vi "Cal.vi"() -> ()   [LabVIEW 2012]
panel:
  in  "3. Next":bool
  out "Next Ind":bool
  out "Memory Responce Hex":string
  out "Return Count":dbl
  out "Memory Responce Char":string
  out "bit 0":bool
  out "bit 1":bool
  out "bit 2":bool
  out "bit 3":bool
  out "bit 4":bool
  out "bit 5":bool
  out "bit 6":bool
  out "bit 7":bool
  out "T command Bytes sent":dbl
  in  "2. Send address and data":bool
  out "Add Ind":bool
  in  "Starting address HEX string":string
  in  "Data HEX string":string[](array[string])
  in  "Enable":bool
  in  "Input buffer size":u32=16384
  out "Number of bytes written":dbl
  in  "Commant Selector":u16(ring)=1 items=["'X' memory write/read test", "'x' device ID", "'Y' eraze the chip", "'Z' read status register", "'P' Write enable", "'T' Write  Add 3 bytes data 1 byte", "'U' Read", "'u' Byte programming En", "'1' Calibration Values"]
  in  "1. Apply Command":bool
  out "Apply Ind":bool
  out "Message":string
  out "RESET USB":bool
  out "Connected to:":string
  in  "baud rate":u32=1200000
  in  "USB Interface Name":refnum<visa-resource-name>="COM3"
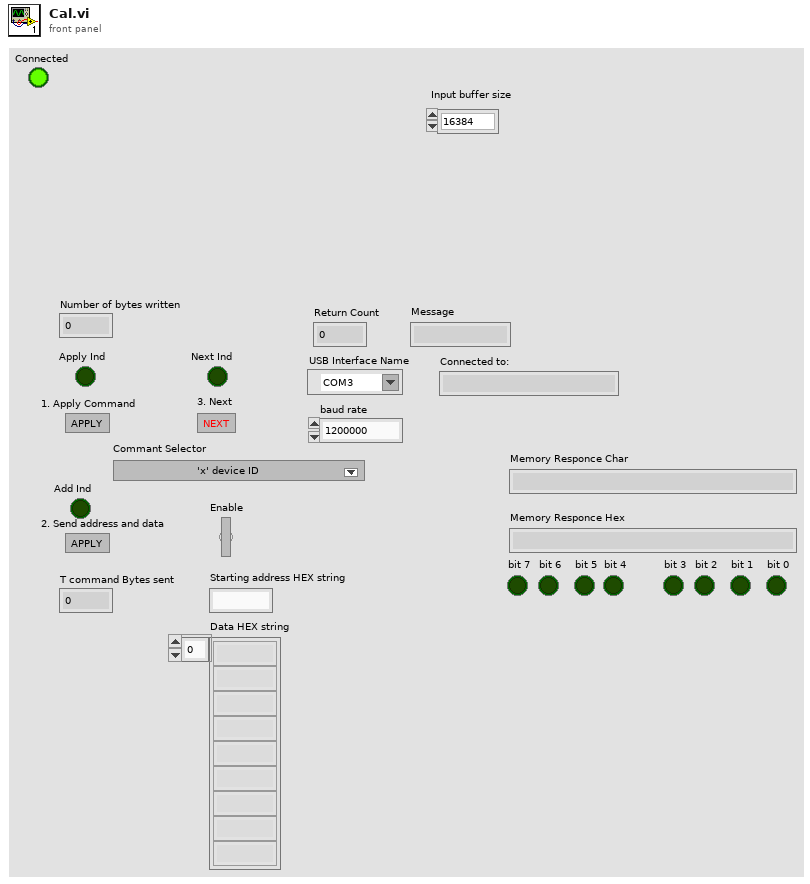
[diagram p1: front panel]
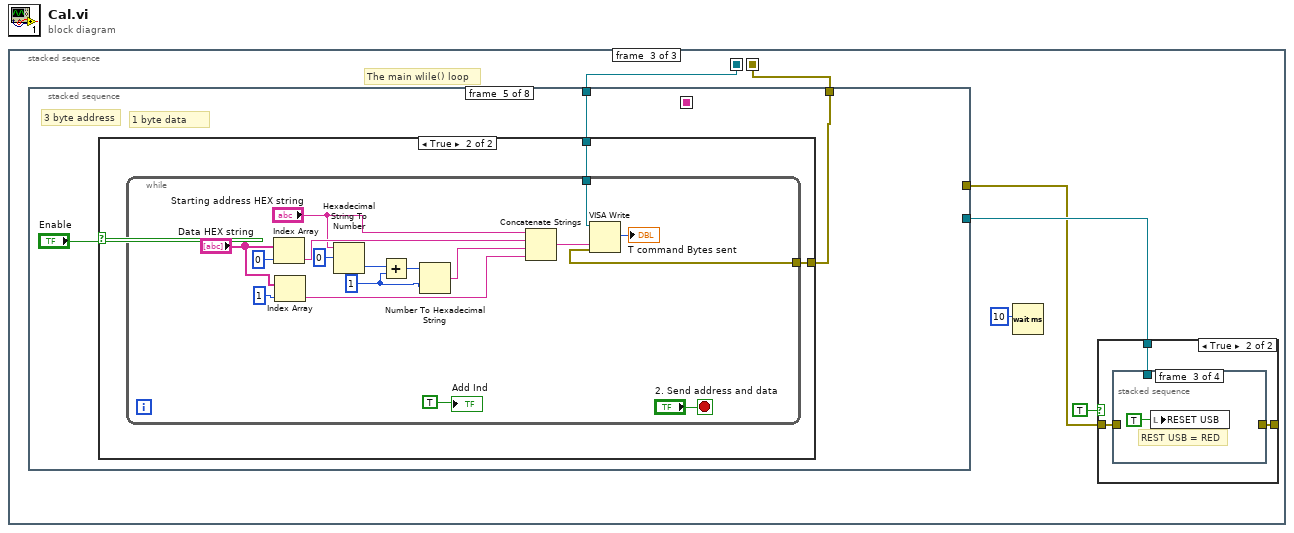
[diagram p0: block diagram]
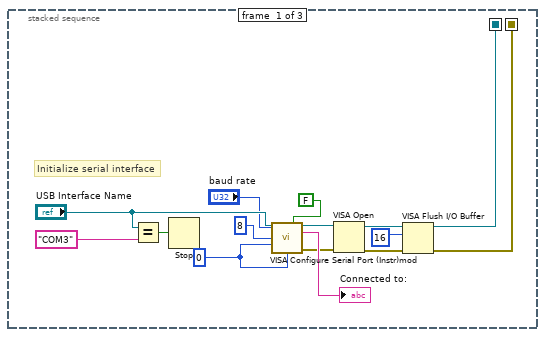
[diagram p2: hidden frame]
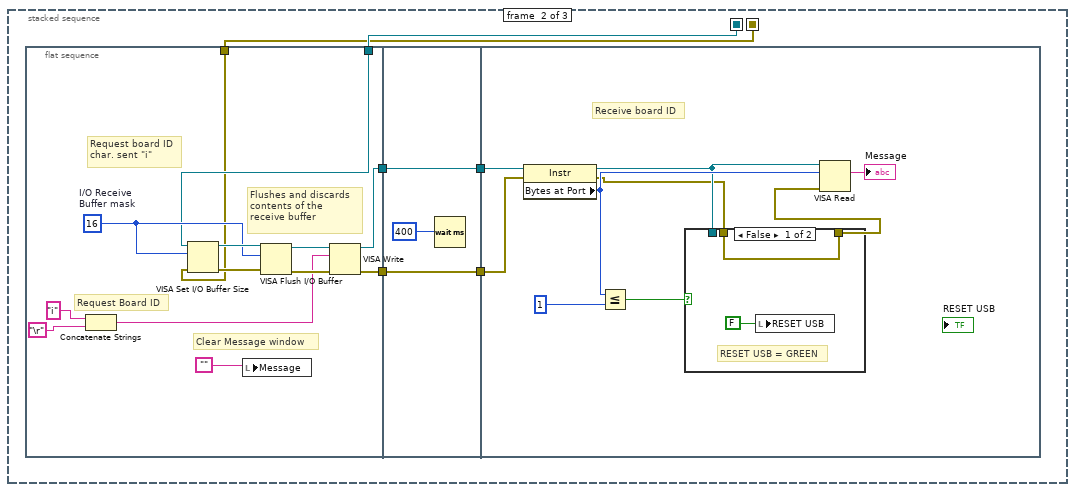
[diagram p3: hidden frame]
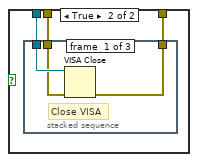
[diagram p4: hidden frame]
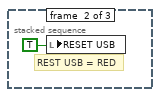
[diagram p5: hidden frame]
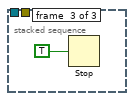
[diagram p6: hidden frame]
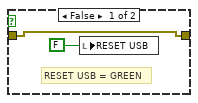
[diagram p7: hidden frame]
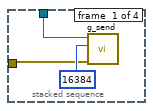
[diagram p8: hidden frame]
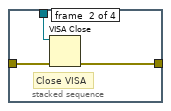
[diagram p9: hidden frame]
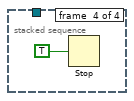
[diagram p10: hidden frame]
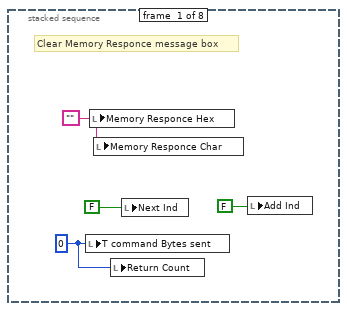
[diagram p11: hidden frame]
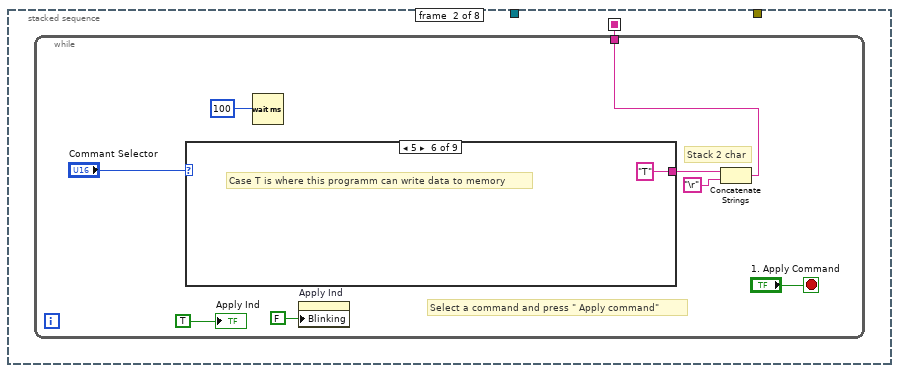
[diagram p12: hidden frame]
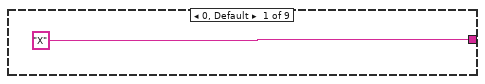
[diagram p13: hidden frame]
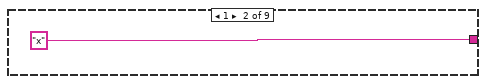
[diagram p14: hidden frame]
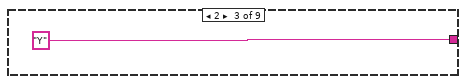
[diagram p15: hidden frame]
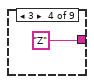
[diagram p16: hidden frame]
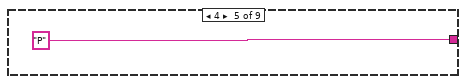
[diagram p17: hidden frame]
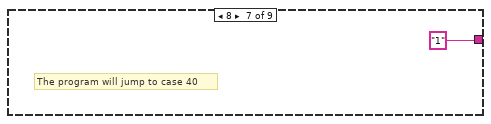
[diagram p18: hidden frame]
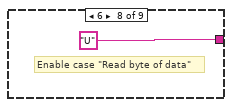
[diagram p19: hidden frame]
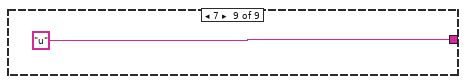
[diagram p20: hidden frame]
diagram:
  n1 = stacked-sequence {
    seq-local: [w2 _ _] -> [_ w16 w61]
    seq-local: [w1 _ _] -> [_ w17 w62]
    frame #0 {
      w4 = 0
      # "Initialize serial interface"
      n2 = Equal?(x="USB Interface Name", y="COM3") -> (x = y?=w14:bool)
      n3 = Stop(stop? (T)=w14) -> ()
      n4 = call "VISA Configure Serial Port (Instr)mod.vi"("VISA resource name"="USB Interface Name", "Enable Termination\nChar (T)"=FALSE, "baud rate (9600)"="baud rate", "data bits (8)"=8, "parity (0:none)"=w4, "flow control (0:none)"=w4) -> ("VISA resource name out"=w8:refnum<visa-resource-name>, "Name"=→"Connected to:":string, "error out"=w7:errorcluster)  [unwired: 6 in, 1 out]
      n5 = VISA Open(error in (no error)=w7, VISA resource name=w8) -> (VISA resource name=w6:refnum<visa-resource-name>, error out=w5:errorcluster)  [unwired: 3 out]
      n6 = VISA Flush I/O Buffer(VISA resource name=w6, mask (16)=u16 16 ("Maskieren (16)"), error in (no error)=w5) -> (VISA resource name out=w1:refnum<visa-resource-name>, error out=w2:errorcluster)
    }
    frame #1 {
      n7 = flat-sequence {
        tunnel: w17 -> [w26]
        tunnel: w16 -> [w25]
        tunnel: [w24] -> w21
        tunnel: [w23] -> w20
        tunnel: [w36] -> w19
        tunnel: w21 -> [w36]
        tunnel: [w35] -> w18
        tunnel: w20 -> [w35]
        tunnel: w19 -> [w39]
        tunnel: w18 -> [w38]
        frame #0 {
          w30 = u16 16  # I/O Receive Buffer mask
          # "Clear Message window"
          # "Request board ID\nchar. sent \"i\""
          # "Request Board ID"
          # "Flushes and discards \ncontents of the \nreceive buffer"
          n8 = Concatenate Strings("i", "\r") -> (w28:string)
          n9 = VISA Set I/O Buffer Size(VISA resource name=w26, mask (16)=w30, error in (no error)=w25) -> (VISA resource name out=w32:refnum<visa-resource-name>, error out=w31:errorcluster)  [unwired: 1 in]
          n10 = local write "Message"("") -> ()
          n11 = VISA Flush I/O Buffer(VISA resource name=w32, mask (16)=w30, error in (no error)=w31) -> (VISA resource name out=w34:refnum<visa-resource-name>, error out=w33:errorcluster)
          n12 = VISA Write(VISA resource name=w34, write buffer=w28, error in (no error)=w33) -> (VISA resource name out=w24:refnum<visa-resource-name>, error out=w23:errorcluster)  [unwired: 1 out]
        }
        frame #1 {
          n13 = Wait (ms)(milliseconds to wait=400) -> ()  [unwired: 1 out]
        }
        frame #2 {
          # "Receive board ID"
          n14 = property class="Instr"(reference=w39, error in=w38) -> (reference out=w43:refnum<visa-resource-name>, error out=w41:errorcluster, "Bytes at Port"=w45:u32)
          n15 = Less Or Equal?(x=w45, y=1) -> (x <= y?=w46:bool)
          n16 = case shown="False" w46 {
            tunnel: w43 -> [_ w51]
            tunnel: w41 -> [w47 w50]
            tunnel: [w47 w49] -> w40
            frame False {
              # "RESET USB = GREEN"
              n17 = local write "RESET USB"(FALSE) -> ()
            }
            frame True {
              n18 = stacked-sequence {
                tunnel: w51 -> [w54 _ _]
                tunnel: w50 -> [w53 _ _]
                tunnel: [w52 _ _] -> w49
                frame #0 {
                  # "Close VISA"
                  n19 = VISA Close(VISA resource name=w54, error in (no error)=w53) -> (error out=w52:errorcluster)
                }
                frame #1 {
                  # "REST USB = RED"
                  n20 = local write "RESET USB"(TRUE) -> ()
                }
                frame #2 {
                  n21 = Stop(stop? (T)=TRUE ("Stop? (T)")) -> ()
                }
              }
            }
          }
          n22 = VISA Read(VISA resource name=w43, byte count=w45, error in (no error)=w40) -> (read buffer=→"Message":string)  [unwired: 3 out]
        }
      }
    }
    frame #2 {
      # "The main wlile() loop"
      n23 = stacked-sequence {
        seq-local: [_ w80 _ _ _ _ _ _] -> [_ _ w101 _ _ _ _ _]
        tunnel: w62 -> [_ _ w103 _ w112 _ w157 _]
        tunnel: w61 -> [_ _ w102 _ w111 _ w159 _]
        tunnel: [_ _ _ _ _ _ w156 _] -> w57
        tunnel: [_ _ _ _ _ _ w154 _] -> w58
        frame #0 {
          w77 = 0
          w79 = ""
          # "Clear Memory Responce message box"
          n24 = local write "T command Bytes sent"(w77) -> ()
          n25 = local write "Memory Responce Hex"(w79) -> ()
          n26 = local write "Memory Responce Char"(w79) -> ()
          n27 = local write "Return Count"(w77) -> ()
          n28 = local write "Next Ind"(FALSE) -> ()
          n29 = local write "Add Ind"(FALSE) -> ()
        }
        frame #1 {
          n30 = while {
            tunnel: [w81] -> w80
            stop <- "1. Apply Command" stop-if-true
            # "Select a command and press \" Apply command\""
            # "Stack 2 char"
            n31 = case shown="5" "Commant Selector" {
              tunnel: ["X" "x" "Y" "Z" "P" "T" "1" "U" "u"] -> w87
              frame 0, Default {
              }
              frame 1 {
              }
              frame 2 {
              }
              frame 3 {
              }
              frame 4 {
              }
              frame 5 {
                # "Case T is where this programm can write data to memory"
              }
              frame 8 {
                # "The program will jump to case 40"
              }
              frame 6 {
                # "Enable case \"Read byte of data\""
              }
              frame 7 {
              }
            }
            n32 = Wait (ms)(milliseconds to wait=100) -> ()  [unwired: 1 out]
            n33 = property on="Apply Ind" class="Bool (strict)"("Blinking"=FALSE) -> ()  [unwired: 2 in, 2 out]
            n34 = Concatenate Strings(w87, "\r") -> (w81:string)
            "Apply Ind" <- TRUE
          }
        }
        frame #2 {
          w104 = u16 16  # I/O Receive Buffer mask
          # "Write command"
          # "Previously selected command is sent to the FB"
          # "Flushes and discards \ncontents of the \nreceive buffer"
          n35 = local write "Apply Ind"(FALSE) -> ()
          n36 = VISA Set I/O Buffer Size(VISA resource name=w103, mask (16)=w104, size (4096)="Input buffer size", error in (no error)=w102) -> (VISA resource name out=w106:refnum<visa-resource-name>, error out=w105:errorcluster)
          n37 = VISA Flush I/O Buffer(VISA resource name=w106, mask (16)=w104, error in (no error)=w105) -> (VISA resource name out=w108:refnum<visa-resource-name>, error out=w107:errorcluster)
          n38 = VISA Write(VISA resource name=w108, write buffer=w101, error in (no error)=w107) -> (return count=→"Number of bytes written":u32)  [unwired: 2 out]
        }
        frame #3 {
          n39 = Wait (ms)(milliseconds to wait=10) -> ()  [unwired: 1 out]
        }
        frame #4 {
          # "1 byte data"
          # "3 byte address"
          n40 = case shown="True" "Enable" {
            tunnel: w112 -> [_ w113]
            tunnel: w111 -> [_ w114]
            frame False {
            }
            frame True {
              n41 = while {
                tunnel: w114 -> [w131]
                tunnel: w113 -> [w130]
                stop <- "2. Send address and data" stop-if-true
                w115 = 1
                n42 = Index Array(array="Data HEX string", index=0) -> (element=w124:string)
                n43 = Index Array(array="Data HEX string", index=1) -> (element=w121:string)
                n44 = Hexadecimal String To Number(string="Starting address HEX string", offset=0) -> (number=w120:u32)  [unwired: 1 in, 1 out]
                n45 = Add(x=w120, y=w115) -> (x+y=w117:u32)
                n46 = Number To Hexadecimal String(1:w115, 2:w117) -> (0:w116:string)
                n47 = Concatenate Strings("Starting address HEX string", w124, w116, w121) -> (w126:string)
                n48 = VISA Write(VISA resource name=w130, write buffer=w126, error in (no error)=w131) -> (return count=→"T command Bytes sent":u32)  [unwired: 2 out]
                "Add Ind" <- TRUE
              }
            }
          }
        }
        frame #5 {
          n49 = Wait (ms)(milliseconds to wait=100) -> ()  [unwired: 1 out]
          n50 = local write "Add Ind"(FALSE) -> ()
        }
        frame #6 {
          n51 = property class="Instr"(reference=w157, error in=w159) -> (reference out=w160:refnum<visa-resource-name>, error out=w158:errorcluster, "Bytes at Port"=w161:u32)
          n52 = VISA Read(VISA resource name=w160, byte count=w161, error in (no error)=w158) -> (VISA resource name out=w154:refnum<visa-resource-name>, read buffer=w136:string, return count=→"Return Count":u32, error out=w156:errorcluster)
          "Memory Responce Hex" <- w136
          "Memory Responce Char" <- w136
          n53 = String To Byte Array(string=w136) -> (unsigned byte array=w135:u8[])
          n54 = Index Array(array=w135) -> (element=w134:u8)  [unwired: 1 in]
          n55 = Number To Boolean Array(number=w134) -> (Boolean array=w141:bool[])
          n56 = Index Array(array=w141, index=1) -> (element=→"bit 1":bool)
          n57 = Index Array(array=w141, index=3) -> (element=→"bit 3":bool)
          n58 = Index Array "Index Array"(array=w141, index=0) -> (element=→"bit 0":bool)
          n59 = Index Array(array=w141, index=2) -> (element=→"bit 2":bool)
          n60 = Index Array(array=w141, index=5) -> (element=→"bit 5":bool)
          n61 = Index Array(array=w141, index=7) -> (element=→"bit 7":bool)
          n62 = Index Array "Index Array"(array=w141, index=4) -> (element=→"bit 4":bool)
          n63 = Index Array(array=w141, index=6) -> (element=→"bit 6":bool)
        }
        frame #7 {
          n64 = while {
            stop <- "3. Next" stop-if-true
            # "This delay allows to view MCU responce"
            n65 = Wait (ms)(milliseconds to wait=100) -> ()  [unwired: 1 out]
            "Next Ind" <- TRUE
          }
        }
      }
      n66 = Wait (ms)(milliseconds to wait=10) -> ()  [unwired: 1 out]
      n67 = case shown="True" TRUE {
        tunnel: w58 -> [_ w67]
        tunnel: w57 -> [w63 w66]
        tunnel: [w63 w65] -> _
        frame False {
          # "RESET USB = GREEN"
          n68 = local write "RESET USB"(FALSE) -> ()
        }
        frame True {
          n69 = stacked-sequence {
            tunnel: w67 -> [w69 w73 _ _]
            tunnel: w66 -> [w68 w72 _ _]
            tunnel: [_ w71 _ _] -> w65
            frame #0 {
              n70 = call "g_send.vi"("error in (no error)"=w68, "Input buffer size"=16384, "USB Interface Name"=w69) -> ()  [unwired: 8 in, 1 out]
            }
            frame #1 {
              # "Close VISA"
              n71 = VISA Close(VISA resource name=w73, error in (no error)=w72) -> (error out=w71:errorcluster)
            }
            frame #2 {
              # "REST USB = RED"
              n72 = local write "RESET USB"(TRUE) -> ()
            }
            frame #3 {
              n73 = Stop(stop? (T)=TRUE ("Stop? (T)")) -> ()
            }
          }
        }
      }
    }
  }
